vi "Interpret Driver Controls.vi"() -> ()   [LabVIEW 2018]
uses:
  SubSystems/Controllers/Driver Controller/Driver Controller Global.vi
  SubSystems/Drive Train/Drive Train Global.vi
  SubSystems/Lift/Lift Global.vi
  SubSystems/Controllers/Manipulator Controlller/Manipulator Controller Global.vi
  SubSystems/Cargo Intake/Cargo Intake Global.vi
  SubSystems/HAB Climber/HAB Climber Global.vi
  SubSystems/Hatch Panel Intake/Hatch Panel Intake Global.vi
  Robot Global Data.vi
  <vilib>/addons/control/pid/NI_PID_pid.lvlib
  <vilib>/addons/control/pid/pid.llb/PID (DBL).vi
panel:
  in  "Auto Pickup Height":dbl=10.0
  in  "Camera Tracking":T1={"proportional gain (Kc)"=1.0, "integral time (Ti, min)"=0.01, "derivative time (Td, min)"=0.0}
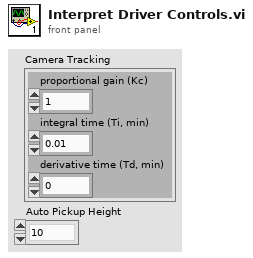
[diagram p1: front panel]
types:
  T1 = cluster{"proportional gain (Kc)":dbl, "integral time (Ti, min)":dbl, "derivative time (Td, min)":dbl}
  T2 = cluster{"Rollover":dbl, "Yaw":dbl, "Cont Yaw":dbl}
  T3 = cluster{"offsetAngle H":dbl, "offsetAngle V":dbl, "area":dbl, "skew":dbl, "validTarget":dbl, "latency":dbl}
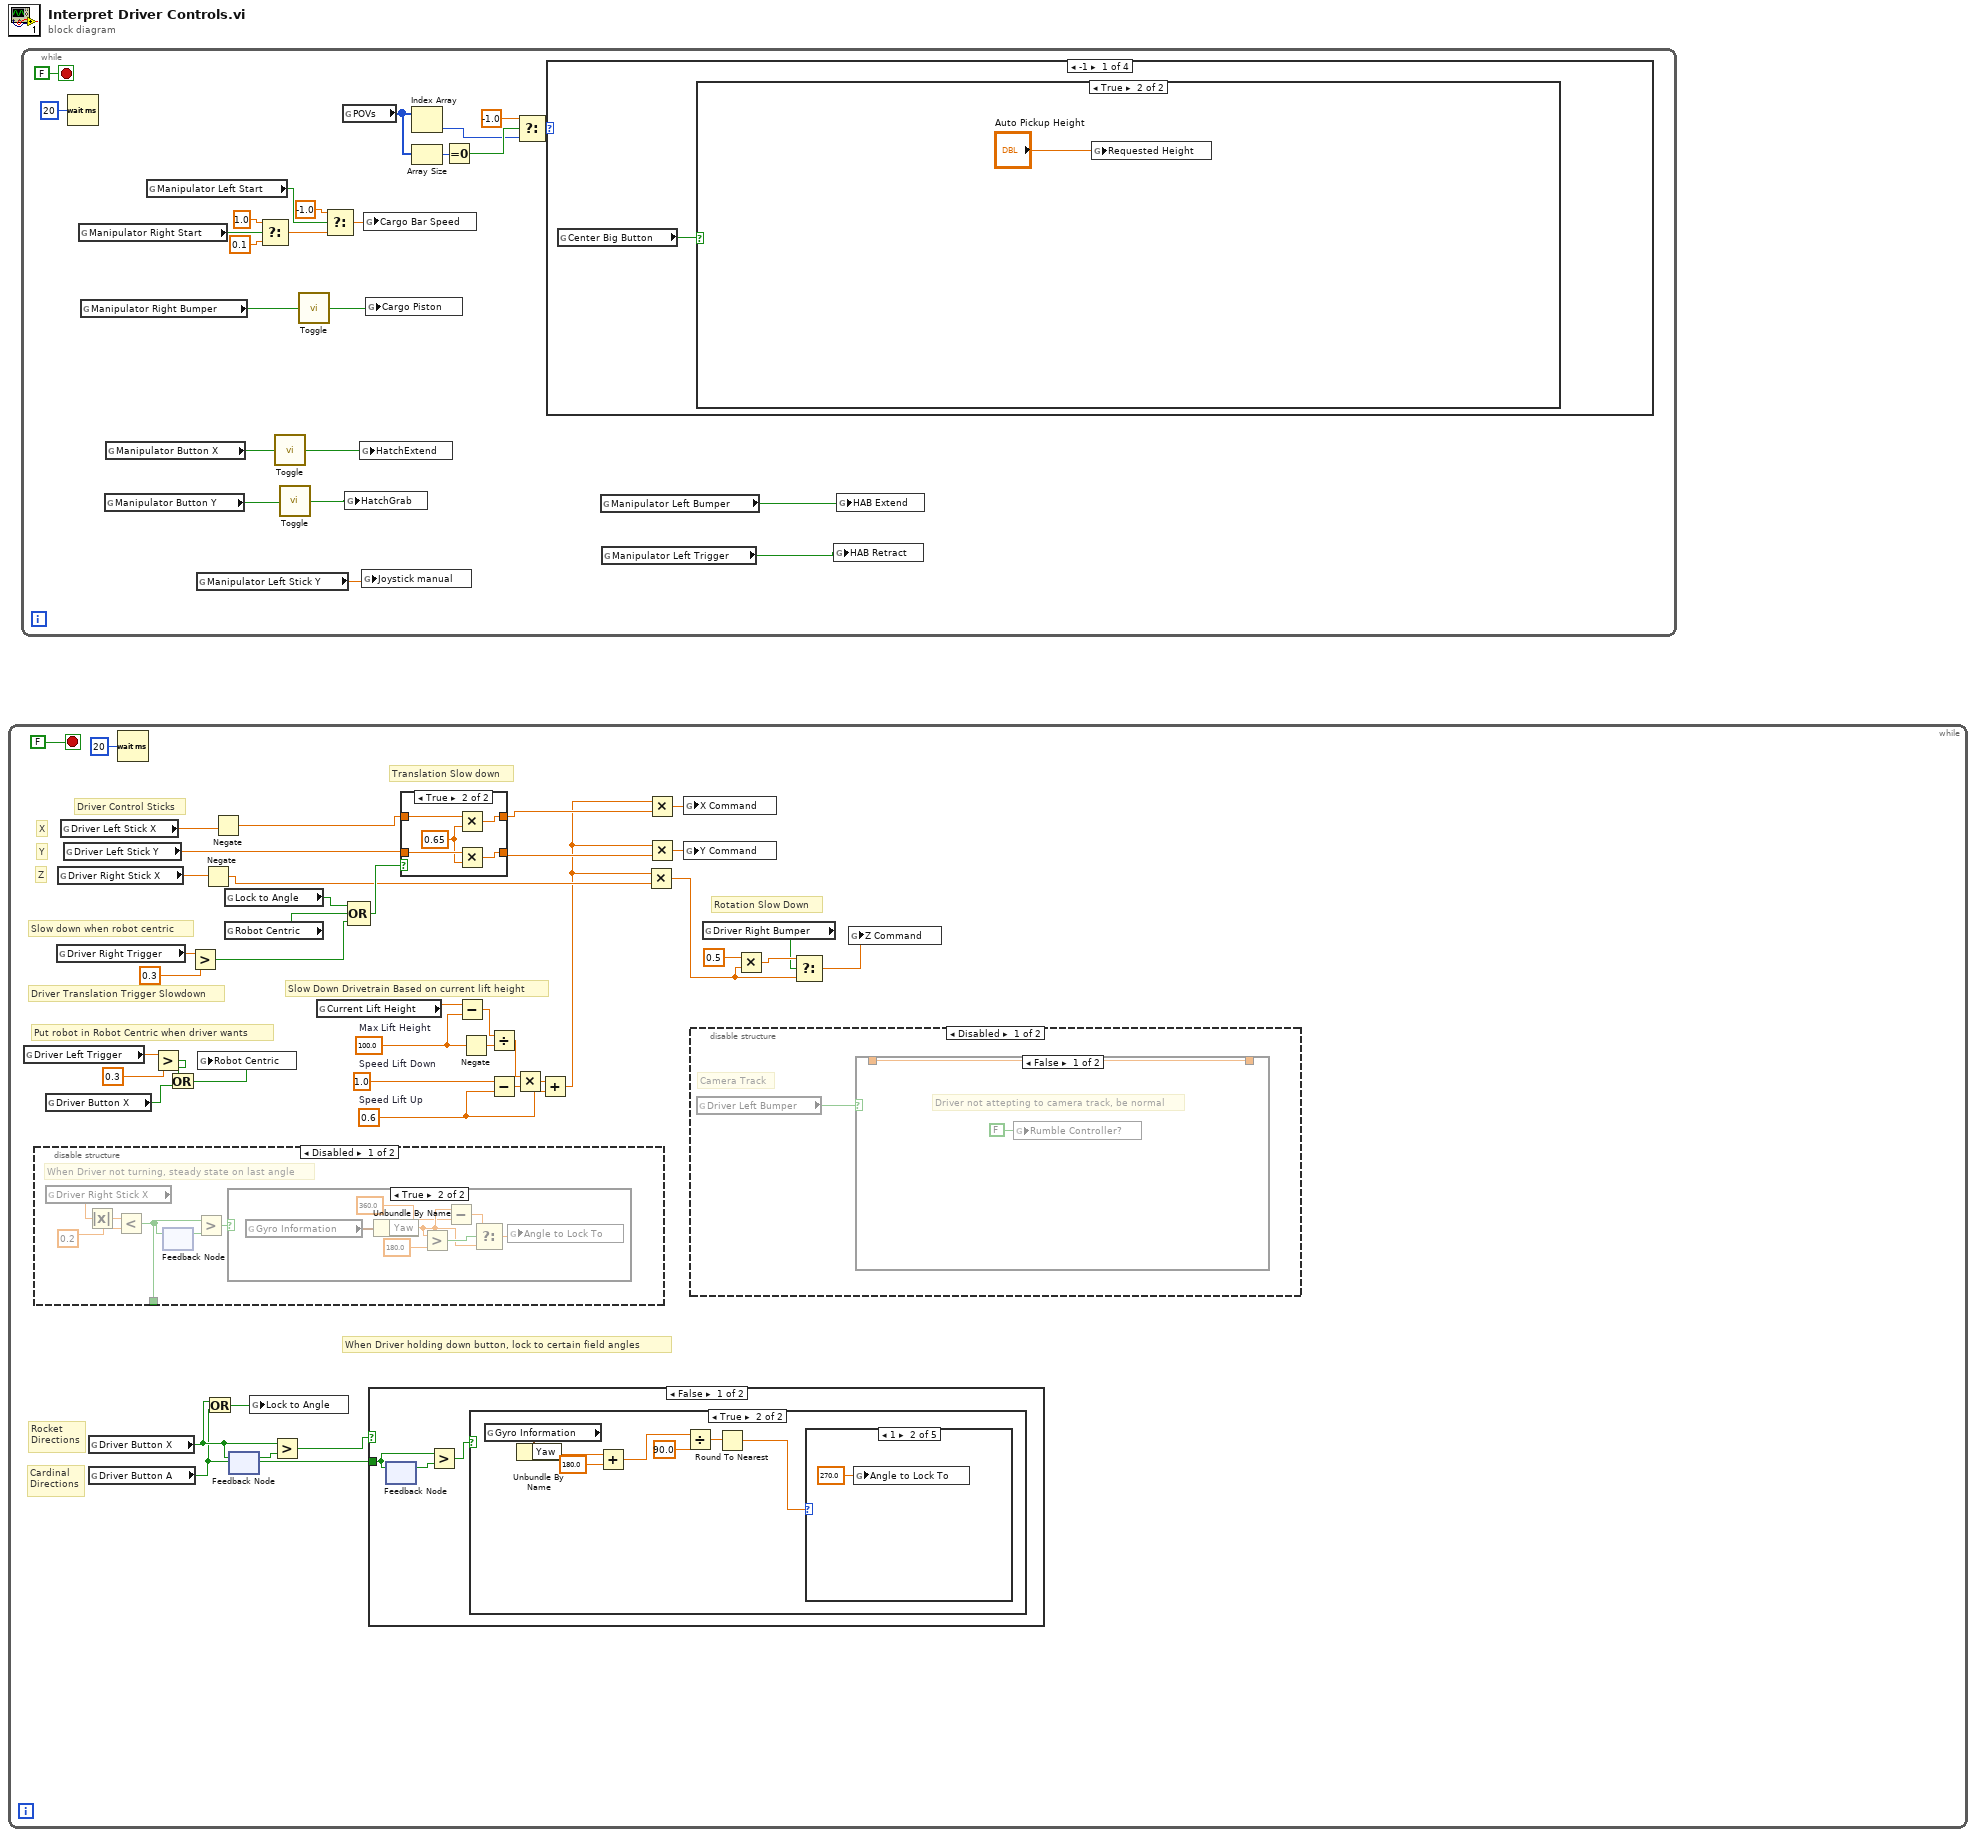
[diagram p0: block diagram]
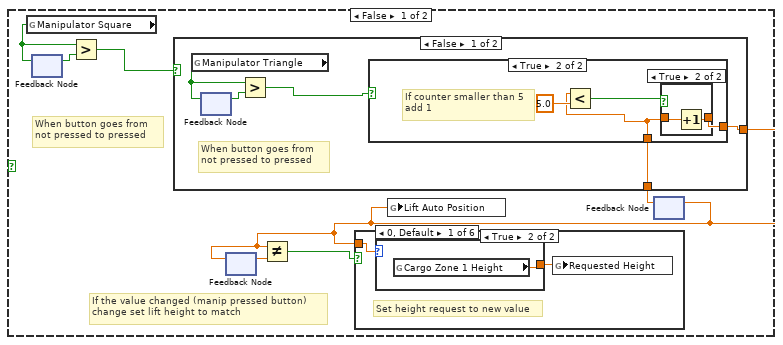
[diagram p2: hidden frame]
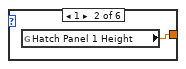
[diagram p4: hidden frame]
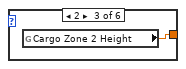
[diagram p5: hidden frame]
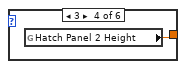
[diagram p6: hidden frame]
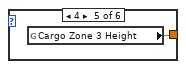
[diagram p7: hidden frame]
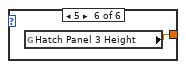
[diagram p8: hidden frame]
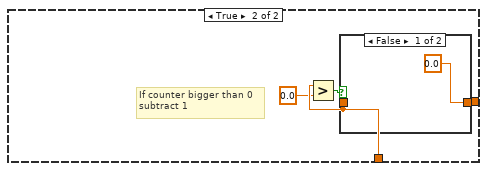
[diagram p11: hidden frame]
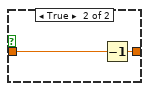
[diagram p12: hidden frame]
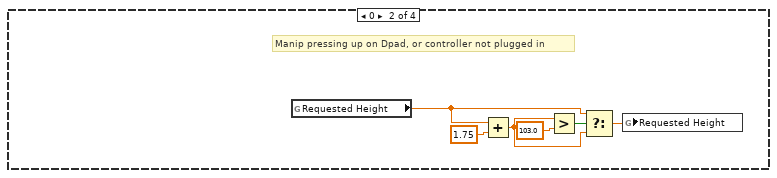
[diagram p13: hidden frame]
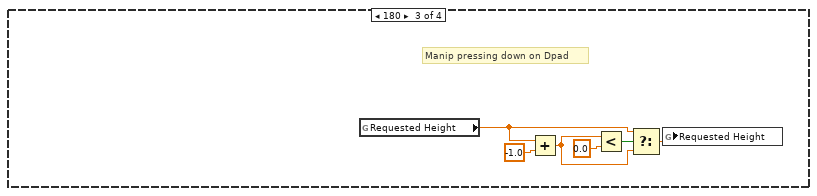
[diagram p14: hidden frame]
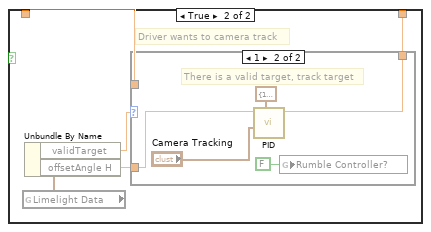
[diagram p16: hidden frame]
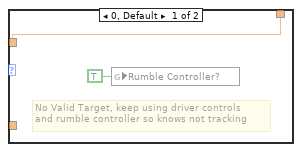
[diagram p17: hidden frame]
diagram:
  n1 = while {
    stop <- FALSE stop-if-true
    w14 = 0.6  # Speed Lift Up
    w18 = 1.0  # Speed Lift Down
    w12 = 100.0  # Max Lift Height
    # "Rotation Slow Down"
    # "Rocket\nDirections"
    # "Cardinal\nDirections"
    # "When Driver holding down button, lock to certain field angles"
    # "Slow Down Drivetrain Based on current lift height"
    # "Put robot in Robot Centric when driver wants"
    # "Slow down when robot centric"
    # "Driver Translation Trigger Slowdown"
    # "Translation Slow down"
    # "Z"
    # "Y"
    # "X"
    # "Driver Control Sticks"
    n2 = global read "Driver Controller Global.vi" "Driver Left Trigger"() -> (w33:dbl)
    n3 = disable-structure shown="Disabled" {
      disable-tunnel: [w58 _] -> _
      frame Disabled {
        # "When Driver not turning, steady state on last angle"
        n4 = global read "Driver Controller Global.vi" "Driver Right Stick X"() -> (w59:dbl)
        n5 = Absolute Value(x=w59) -> (abs(x)=w63:dbl)
        n6 = Less?(x=w63, y=0.2) -> (x < y?=w58:bool)
        n7 = feedback #1() -> (w61:bool)  [unwired: 1 in]
        n8 = feedback-in #1(w58) -> ()
        n9 = Greater?(x=w58, y=w61) -> (0:w60:bool)
        n10 = case shown="True" w60 {
          frame False {
          }
          frame True {
            n11 = global read "Drive Train Global.vi" "Gyro Information"() -> (w70:T2)
            n12 = Unbundle By Name(w70) -> ("Yaw"=w67:dbl)
            n13 = Greater?(x=w67, y=180.0) -> (0:w68:bool)
            n14 = Subtract(x=w67, y=360.0) -> (x-y=w65:dbl)
            n15 = Select(t=w65, s=w68, f=w67) -> (s? t:f=w64:dbl)
            n16 = global write "Drive Train Global.vi" "Angle to Lock To"(w64) -> ()
          }
        }
      }
      frame Enabled {
      }
    }
    n17 = global read "Driver Controller Global.vi" "Driver Button X"() -> (w4:bool)
    n18 = global read "Driver Controller Global.vi" "Driver Right Trigger"() -> (w38:dbl)
    n19 = global read "Driver Controller Global.vi" "Driver Right Stick X"() -> (w39:dbl)
    n20 = global read "Driver Controller Global.vi" "Driver Left Stick X"() -> (w40:dbl)
    n21 = global read "Driver Controller Global.vi" "Driver Left Stick Y"() -> (w21:dbl)
    n22 = global read "Driver Controller Global.vi" "Driver Button X"() -> (w9:bool)
    n23 = global read "Driver Controller Global.vi" "Driver Button A"() -> (w7:bool)
    n24 = Wait (ms)(milliseconds to wait=u32 20) -> ()  [unwired: 1 out]
    n25 = Greater?(x=w33, y=0.3) -> (0:w5:bool)
    n26 = Or(x=w5, y=w4) -> (x .or. y?=w1:bool)
    n27 = Greater?(x=w38, y=0.3) -> (0:w28:bool)
    n28 = global write "Drive Train Global.vi" "Robot Centric"(w1) -> ()
    n29 = Negate(x=w39) -> (-x=w25:dbl)
    n30 = Or(x=w9, y=w7) -> (x .or. y?=w6:bool)
    n31 = Negate(x=w40) -> (-x=w22:dbl)
    n32 = global read "Drive Train Global.vi" "Lock to Angle"() -> (w3:bool)
    n33 = global read "Drive Train Global.vi" "Robot Centric"() -> (w27:bool)
    n34 = feedback #2() -> (w10:bool)  [unwired: 1 in]
    n35 = feedback-in #2(w9) -> ()
    n36 = global write "Drive Train Global.vi" "Lock to Angle"(w6) -> ()
    n37 = Greater?(x=w9, y=w10) -> (0:w8:bool)
    n38 = global read "Lift Global.vi" "Current Lift Height"() -> (w20:dbl)
    n39 = Compound Arithmetic op=OR(w3, w27, w28) -> (w26:bool)
    n40 = case shown="False" w8 {
      tunnel: w7 -> [w72 _]
      frame False {
        n41 = feedback #3() -> (w73:bool)  [unwired: 1 in]
        n42 = feedback-in #3(w72) -> ()
        n43 = Greater?(x=w72, y=w73) -> (0:w71:bool)
        n44 = case shown="True" w71 {
          frame False {
          }
          frame True {
            n45 = global read "Drive Train Global.vi" "Gyro Information"() -> (w80:T2)
            n46 = Unbundle By Name(w80) -> ("Yaw"=w77:dbl)
            n47 = Add(x=w77, y=180.0) -> (x+y=w76:dbl)
            n48 = Divide(x=w76, y=90.0) -> (x/y=w78:dbl)
            n49 = Round To Nearest(number=w78) -> (nearest integer value=w74:dbl)
            n50 = case shown="1" w74 {
              frame 0, Default {
                n51 = global write "Drive Train Global.vi" "Angle to Lock To"(180.0 ("Angle to Lock To")) -> ()
              }
              frame 1 {
                n52 = global write "Drive Train Global.vi" "Angle to Lock To"(270.0 ("Angle to Lock To")) -> ()
              }
              frame 2 {
                n53 = global write "Drive Train Global.vi" "Angle to Lock To"(0.0 ("Angle to Lock To")) -> ()
              }
              frame 3 {
                n54 = global write "Drive Train Global.vi" "Angle to Lock To"(90.0 ("Angle to Lock To")) -> ()
              }
              frame 4 {
                n55 = global write "Drive Train Global.vi" "Angle to Lock To"(180.0 ("Angle to Lock To")) -> ()
              }
            }
          }
        }
      }
      frame True {
        n56 = global read "Drive Train Global.vi" "Gyro Information"() -> (w94:T2)
        n57 = Unbundle By Name(w94) -> ("Cont Yaw"=w92:dbl)
        n58 = Quotient & Remainder(x=w92, y=360.0) -> (x-y*floor(x/y)=w90:dbl)  [unwired: 1 out]
        n59 = Divide(x=w90, y=60.0) -> (x/y=w86:dbl)
        n60 = In Range and Coerce(upper limit=1.5, x=w86, lower limit=0.0) -> (In Range?=w87:bool)  [unwired: 1 out]
        n61 = case shown="False" w87 {
          tunnel: w86 -> [w95 _]
          frame False {
            n62 = In Range and Coerce(upper limit=3.0, x=w95, lower limit=1.5) -> (In Range?=w96:bool)  [unwired: 1 out]
            n63 = case shown="False" w96 {
              tunnel: w95 -> [w101 _]
              tunnel: w95 -> [w99 _]
              frame False {
                n64 = In Range and Coerce(upper limit=4.5, x=w101, lower limit=3.0) -> (In Range?=w100:bool)  [unwired: 1 out]
                n65 = case shown="False" w100 {
                  tunnel: w99 -> [w105 _]
                  frame False {
                    n66 = In Range and Coerce(upper limit=6.0, x=w105, lower limit=4.5) -> (In Range?=w104:bool)  [unwired: 1 out]
                    n67 = case shown="True" w104 {
                      frame False {
                      }
                      frame True {
                        n68 = global write "Drive Train Global.vi" "Angle to Lock To"(330.0 ("Angle to Lock To")) -> ()
                      }
                    }
                  }
                  frame True {
                    n69 = global write "Drive Train Global.vi" "Angle to Lock To"(210.0 ("Angle to Lock To")) -> ()
                  }
                }
              }
              frame True {
                n70 = global write "Drive Train Global.vi" "Angle to Lock To"(150.0 ("Angle to Lock To")) -> ()
              }
            }
          }
          frame True {
            n71 = global write "Drive Train Global.vi" "Angle to Lock To"(30.0 ("Angle to Lock To")) -> ()
          }
        }
      }
    }
    n72 = case shown="True" w26 {
      tunnel: w21 -> [w113 w118]
      tunnel: [w113 w117] -> w24
      tunnel: [w112 w116] -> w23
      tunnel: w22 -> [w112 w115]
      frame False {
      }
      frame True {
        w114 = 0.65 ("Y Slower")
        n73 = Multiply(x=w115, y=w114) -> (x*y=w116:dbl)
        n74 = Multiply(x=w118, y=w114) -> (x*y=w117:dbl)
      }
    }
    n75 = Subtract(x=w20, y=w12) -> (x-y=w19:dbl)
    n76 = Negate(x=w12) -> (-x=w13:dbl)
    n77 = Divide(x=w19, y=w13) -> (x/y=w17:dbl)
    n78 = Subtract(x=w18, y=w14) -> (x-y=w16:dbl)
    n79 = Multiply(x=w17, y=w16) -> (x*y=w15:dbl)
    n80 = Add(x=w15, y=w14) -> (x+y=w11:dbl)
    n81 = Multiply(x=w11, y=w25) -> (x*y=w32:dbl)
    n82 = Multiply(x=w11, y=w23) -> (x*y=w36:dbl)
    n83 = Multiply(x=w11, y=w24) -> (x*y=w35:dbl)
    n84 = global write "Drive Train Global.vi" "X Command"(w36) -> ()
    n85 = global write "Drive Train Global.vi" "Y Command"(w35) -> ()
    n86 = disable-structure shown="Disabled" {
      frame Disabled {
        # "Camera Track"
        n87 = global read "Driver Controller Global.vi" "Driver Left Bumper"() -> (w43:bool)
        n88 = case shown="False" w43 {
          tunnel: _ -> [w45 w48]
          tunnel: [w45 w47] -> _
          frame False {
            # "Driver not attepting to camera track, be normal"
            n89 = global write "Driver Controller Global.vi" "Rumble Controller?"(FALSE ("Rumble Controller?")) -> ()
          }
          frame True {
            # "Driver wants to camera track"
            n90 = global read "Robot Global Data.vi" "Limelight Data"() -> (w50:T3)
            n91 = Unbundle By Name(w50) -> ("validTarget"=w49:dbl, "offsetAngle H"=w46:dbl)
            n92 = case shown="1" w49 {
              tunnel: w48 -> [w52 _]
              tunnel: [w52 w57] -> w47
              tunnel: w46 -> [_ w53]
              frame 0, Default {
                # "No Valid Target, keep using driver controls\nand rumble controller so knows not tracking"
                n93 = global write "Driver Controller Global.vi" "Rumble Controller?"(TRUE ("Rumble Controller?")) -> ()
              }
              frame 1 {
                # "There is a valid target, track target"
                n94 = call-poly <vilib>:"PID.vi"("output range"=cluster{"output high":dbl, "output low":dbl} {"output high"=1.0, "output low"=-1.0}, "PID gains"="Camera Tracking", "setpoint"=w53) -> ("output"=w57:dbl)  [unwired: 7 in, 1 out]
                n95 = global write "Driver Controller Global.vi" "Rumble Controller?"(FALSE ("Rumble Controller?")) -> ()
              }
            }
          }
        }
      }
      frame Enabled {
      }
    }
    n96 = global read "Driver Controller Global.vi" "Driver Right Bumper"() -> (w29:bool)
    n97 = Multiply(x=0.5, y=w32) -> (x*y=w31:dbl)
    n98 = Select(t=w31, s=w29, f=w32) -> (s? t:f=w2:dbl)
    n99 = global write "Drive Train Global.vi" "Z Command"(w2) -> ()
  }
  n100 = while {
    stop <- FALSE stop-if-true
    n101 = Wait (ms)(milliseconds to wait=u32 20) -> ()  [unwired: 1 out]
    n102 = global read "Manipulator Controller Global.vi" "Manipulator Right Start"() -> (w137:bool)
    n103 = global read "Manipulator Controller Global.vi" "Manipulator Right Bumper"() -> (w140:bool)
    n104 = global read "Manipulator Controller Global.vi" "Manipulator Button Y"() -> (w131:bool)
    n105 = global read "Manipulator Controller Global.vi" "Manipulator Button X"() -> (w129:bool)
    n106 = global read "Manipulator Controller Global.vi" "Manipulator Left Start"() -> (w136:bool)
    n107 = global read "Manipulator Controller Global.vi" "Manipulator Left Stick Y"() -> (w121:dbl)
    n108 = Select(t=1.0, s=w137, f=0.1) -> (s? t:f=w135:dbl)
    n109 = call "Toggle.vi"("Input"=w129) -> ("Output"=w130:bool)
    n110 = call "Toggle.vi"("Input"=w131) -> ("Output"=w122:bool)
    n111 = call "Toggle.vi"("Input"=w140) -> ("Output"=w139:bool)
    n112 = Select(t=-1.0, s=w136, f=w135) -> (s? t:f=w138:dbl)
    n113 = global read "Manipulator Controller Global.vi" "POVs"() -> (w128:i16[])
    n114 = global write "Hatch Panel Intake Global.vi" "HatchGrab"(w122) -> ()
    n115 = global write "Hatch Panel Intake Global.vi" "HatchExtend"(w130) -> ()
    n116 = global write "Lift Global.vi" "Joystick manual"(w121) -> ()
    n117 = global write "Cargo Intake Global.vi" "Cargo Bar Speed"(w138) -> ()
    n118 = global write "Cargo Intake Global.vi" "Cargo Piston"(w139) -> ()
    n119 = Index Array(array=w128) -> (element=w123:i16)  [unwired: 1 in]
    n120 = Array Size(array=w128) -> (size(s)=w127:i32)
    n121 = Equal To 0?(x=w127) -> (x = 0?=w125:bool)
    n122 = Select(t=-1.0, s=w125, f=w123) -> (s? t:f=w126:dbl)
    n123 = case shown="-1" w126 {
      frame -1 {
        n124 = global read "Manipulator Controller Global.vi" "Center Big Button"() -> (w143:bool)
        n125 = case shown="True" w143 {
          frame False {
            # "If the value changed (manip pressed button)\nchange set lift height to match"
            # "When button goes from\nnot pressed to pressed"
            n126 = global read "Manipulator Controller Global.vi" "Manipulator Square"() -> (w149:bool)
            n127 = feedback #4() -> (w150:bool)  [unwired: 1 in]
            n128 = feedback-in #4(w149) -> ()
            n129 = Greater?(x=w149, y=w150) -> (0:w146:bool)
            n130 = feedback #5() -> (w144:dbl)  [unwired: 1 in]
            n131 = feedback #6() -> (w148:dbl)  [unwired: 1 in]
            n132 = case shown="False" w146 {
              tunnel: [w160 w175] -> w145
              tunnel: w148 -> [w161 w174]
              frame False {
                # "When button goes from\nnot pressed to pressed"
                n133 = global read "Manipulator Controller Global.vi" "Manipulator Triangle"() -> (w163:bool)
                n134 = feedback #7() -> (w162:bool)  [unwired: 1 in]
                n135 = feedback-in #7(w163) -> ()
                n136 = Greater?(x=w163, y=w162) -> (0:w159:bool)
                n137 = case shown="True" w159 {
                  tunnel: w161 -> [w164 w166]
                  tunnel: [w164 w168] -> w160
                  frame False {
                  }
                  frame True {
                    # "If counter smaller than 5\nadd 1"
                    n138 = Less?(x=w166, y=5.0) -> (x < y?=w165:bool)
                    n139 = case shown="True" w165 {
                      tunnel: [w169 w171] -> w168
                      tunnel: w166 -> [w169 w170]
                      frame False {
                      }
                      frame True {
                        n140 = Increment(x=w170) -> (x+1=w171:dbl)
                      }
                    }
                  }
                }
              }
              frame True {
                # "If counter bigger than 0\nsubtract 1"
                n141 = Greater?(x=w174, y=0.0) -> (0:w173:bool)
                n142 = case shown="False" w173 {
                  tunnel: [0.0 ("y") w178] -> w175
                  tunnel: w174 -> [_ w177]
                  frame False {
                  }
                  frame True {
                    n143 = Decrement(x=w177) -> (x-1=w178:dbl)
                  }
                }
              }
            }
            n144 = feedback-in #5(w145) -> ()
            n145 = Not Equal?(x=w145, y=w144) -> (x != y?=w147:bool)
            n146 = case shown="True" w147 {
              tunnel: w145 -> [_ w151]
              frame False {
                # "Manipulator didnt request change"
              }
              frame True {
                # "Set height request to new value"
                n147 = case shown="0, Default" w151 {
                  tunnel: [w153 w154 w155 w156 w157 w158] -> w152
                  frame 0, Default {
                    n148 = global read "Lift Global.vi" "Cargo Zone 1 Height"() -> (w153:dbl)
                  }
                  frame 1 {
                    n149 = global read "Lift Global.vi" "Hatch Panel 1 Height"() -> (w154:dbl)
                  }
                  frame 2 {
                    n150 = global read "Lift Global.vi" "Cargo Zone 2 Height"() -> (w155:dbl)
                  }
                  frame 3 {
                    n151 = global read "Lift Global.vi" "Hatch Panel 2 Height"() -> (w156:dbl)
                  }
                  frame 4 {
                    n152 = global read "Lift Global.vi" "Cargo Zone 3 Height"() -> (w157:dbl)
                  }
                  frame 5 {
                    n153 = global read "Lift Global.vi" "Hatch Panel 3 Height"() -> (w158:dbl)
                  }
                }
                n154 = global write "Lift Global.vi" "Requested Height"(w152) -> ()
              }
            }
            n155 = global write "Lift Global.vi" "Lift Auto Position"(w145) -> ()
            n156 = feedback-in #6(w145) -> ()
          }
          frame True {
            n157 = global write "Lift Global.vi" "Requested Height"("Auto Pickup Height") -> ()
          }
        }
      }
      frame 0 {
        # "Manip pressing up on Dpad, or controller not plugged in"
        n158 = global read "Lift Global.vi" "Requested Height"() -> (w181:dbl)
        n159 = Add(x=w181, y=1.75) -> (x+y=w180:dbl)
        n160 = Greater?(x=w180, y=103.0) -> (0:w182:bool)
        n161 = Select(t=w181, s=w182, f=w180) -> (s? t:f=w183:dbl)
        n162 = global write "Lift Global.vi" "Requested Height"(w183) -> ()
      }
      frame 180 {
        # "Manip pressing down on Dpad"
        n163 = global read "Lift Global.vi" "Requested Height"() -> (w186:dbl)
        n164 = Add(x=w186, y=-1.0) -> (x+y=w188:dbl)
        n165 = Less?(x=w188, y=0.0) -> (x < y?=w189:bool)
        n166 = Select(t=w186, s=w189, f=w188) -> (s? t:f=w187:dbl)
        n167 = global write "Lift Global.vi" "Requested Height"(w187) -> ()
      }
      frame -100, Default {
      }
    }
    n168 = global read "Manipulator Controller Global.vi" "Manipulator Left Bumper"() -> (w120:bool)
    n169 = global read "Manipulator Controller Global.vi" "Manipulator Left Trigger"() -> (w119:bool)
    n170 = global write "HAB Climber Global.vi" "HAB Retract"(w119) -> ()
    n171 = global write "HAB Climber Global.vi" "HAB Extend"(w120) -> ()
  }
